vi "Cargo State Machine.vi"() -> (0 "Cargo Intake Bar":dbl, 3 "Cargo Piston":bool)   [LabVIEW 2018]
uses:
  SubSystems/Cargo Intake/Cargo Intake Global.vi
panel:
  in  "Boolean 2":bool
  in  "Boolean":bool
  out "Numeric":dbl
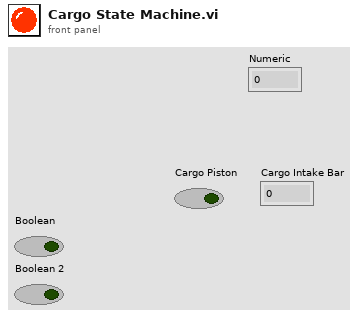
[diagram p1: front panel]
types:
  T1 = enum16{"Up + No Cargo", "Move Down", "Down + Intake", "Move Up", "Up + Cargo"}
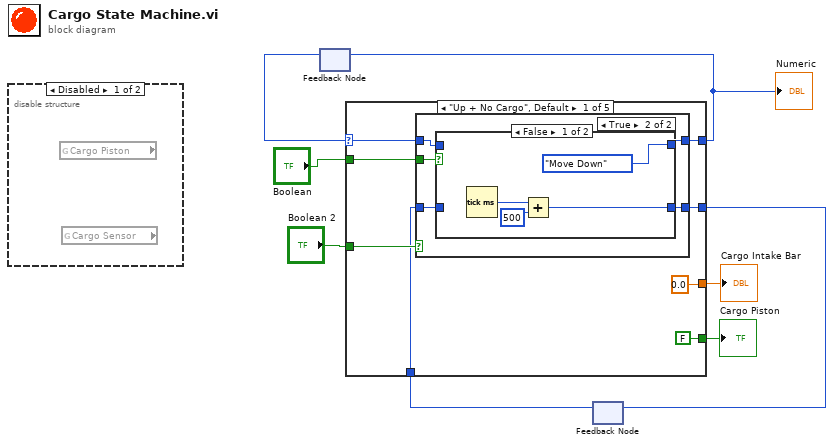
[diagram p0: block diagram]
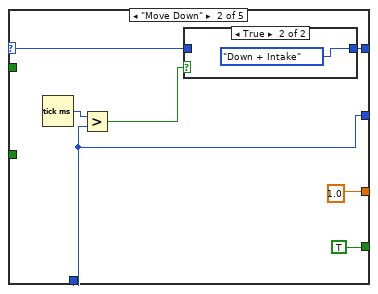
[diagram p5: hidden frame]
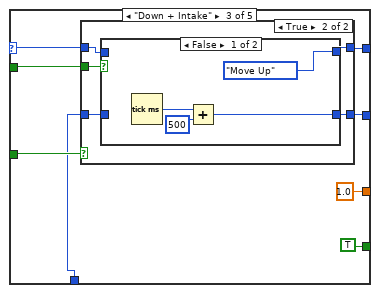
[diagram p7: hidden frame]
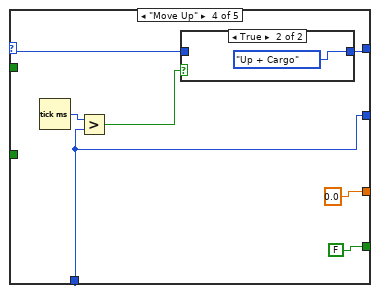
[diagram p10: hidden frame]
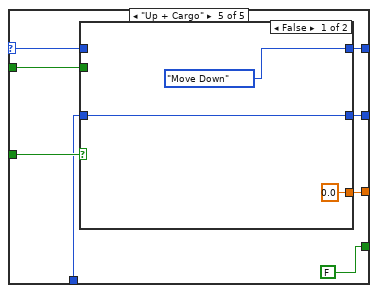
[diagram p12: hidden frame]
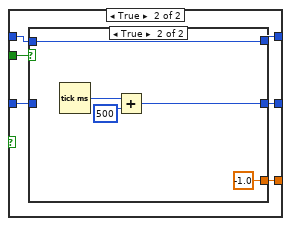
[diagram p13: hidden frame]
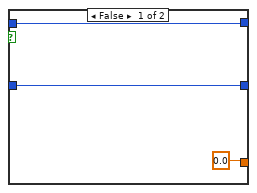
[diagram p14: hidden frame]
diagram:
  n1 = disable-structure shown="Disabled" {
    frame Disabled {
      n2 = global read "Cargo Intake Global.vi" "Cargo Piston"() -> ()  [unwired: 1 out]
      n3 = global read "Cargo Intake Global.vi" "Cargo Sensor"() -> ()  [unwired: 1 out]
    }
    frame Enabled {
    }
  }
  n4 = feedback #1() -> (w8:T1)  [unwired: 1 in]
  n5 = feedback #2() -> (w4:u32)  [unwired: 1 in]
  n6 = case shown="\"Up + No Cargo\", Default" w8 {
    selector: w8 -> [w14 w35 w44 w62 w74]
    tunnel: [w16 w36 w43 w64 w73] -> w3
    tunnel: "Boolean" -> [w15 _ w45 _ w75]
    tunnel: [FALSE TRUE TRUE FALSE FALSE] -> w7
    tunnel: [0.0 1.0 1.0 0.0 w71] -> w6
    tunnel: "Boolean 2" -> [w11 _ w46 _ w76]
    tunnel: [w10 w32 w42 w60 w72] -> w5
    tunnel: w4 -> [w9 w32 w39 w60 w69]
    frame "Up + No Cargo", Default {
      n7 = case shown="False" w11 {
        tunnel: [w21 w29] -> w16
        tunnel: w15 -> [w20 _]
        tunnel: w14 -> [w19 w29]
        tunnel: [w18 w28] -> w10
        tunnel: w9 -> [w17 w28]
        frame False {
          n8 = case shown="True" w20 {
            tunnel: [w23 T1."Move Down" ("Enum")] -> w21
            tunnel: w19 -> [w23 _]
            tunnel: [w22 w24] -> w18
            tunnel: w17 -> [w22 _]
            frame False {
            }
            frame True {
              n9 = Tick Count (ms)() -> (millisecond timer value=w26:u32)
              n10 = Add(x=w26, y=u32 500) -> (x+y=w24:u32)
            }
          }
        }
        frame True {
        }
      }
    }
    frame "Move Down" {
      n11 = Tick Count (ms)() -> (millisecond timer value=w34:u32)
      n12 = Greater?(x=w34, y=w32) -> (0:w33:bool)
      n13 = case shown="True" w33 {
        tunnel: [w37 T1."Down + Intake" ("Enum")] -> w36
        tunnel: w35 -> [w37 _]
        frame False {
        }
        frame True {
        }
      }
    }
    frame "Down + Intake" {
      n14 = case shown="True" w46 {
        tunnel: [w48 w53] -> w43
        tunnel: w45 -> [_ w52]
        tunnel: w44 -> [w48 w51]
        tunnel: [w47 w50] -> w42
        tunnel: w39 -> [w47 w49]
        frame False {
        }
        frame True {
          n15 = case shown="False" w52 {
            tunnel: [T1."Move Up" ("Enum") w59] -> w53
            tunnel: w51 -> [_ w59]
            tunnel: [w54 w58] -> w50
            tunnel: w49 -> [_ w58]
            frame False {
              n16 = Tick Count (ms)() -> (millisecond timer value=w56:u32)
              n17 = Add(x=w56, y=u32 500) -> (x+y=w54:u32)
            }
            frame True {
            }
          }
        }
      }
    }
    frame "Move Up" {
      n18 = Tick Count (ms)() -> (millisecond timer value=w65:u32)
      n19 = Greater?(x=w65, y=w60) -> (0:w66:bool)
      n20 = case shown="True" w66 {
        tunnel: [w67 T1."Up + Cargo" ("Enum")] -> w64
        tunnel: w62 -> [w67 _]
        frame False {
        }
        frame True {
        }
      }
    }
    frame "Up + Cargo" {
      n21 = case shown="False" w76 {
        tunnel: [T1."Move Down" ("Enum") w85] -> w73
        tunnel: w75 -> [_ w84]
        tunnel: w74 -> [_ w83]
        tunnel: [w79 w82] -> w72
        tunnel: w69 -> [w79 w81]
        tunnel: [0.0 w80] -> w71
        frame False {
        }
        frame True {
          n22 = case shown="True" w84 {
            tunnel: [w88 w89] -> w85
            tunnel: w83 -> [w88 w89]
            tunnel: [w87 w91] -> w82
            tunnel: w81 -> [w87 _]
            tunnel: [0.0 -1.0] -> w80
            frame False {
            }
            frame True {
              n23 = Tick Count (ms)() -> (millisecond timer value=w93:u32)
              n24 = Add(x=w93, y=u32 500) -> (x+y=w91:u32)
            }
          }
        }
      }
    }
  }
  "Cargo Intake Bar" <- w6
  "Cargo Piston" <- w7
  "Numeric" <- w3
  n25 = feedback-in #1(w3) -> ()
  n26 = feedback-in #2(w5) -> ()
